vi "sub_qam_demod.vi"(8 "symbol map":cdb[](array[numeric]), 11 "symbol":cdb[](array[numeric])) -> (3 "bitstream":i16[](array[numeric]))   [LabVIEW 2014]
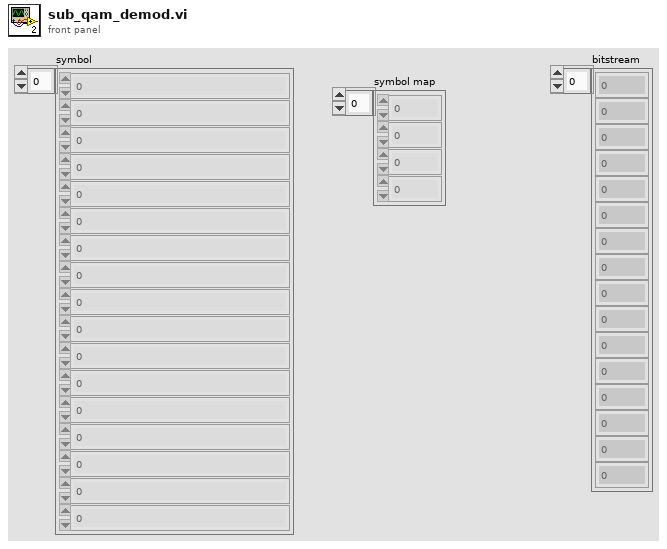
[diagram p1: front panel]
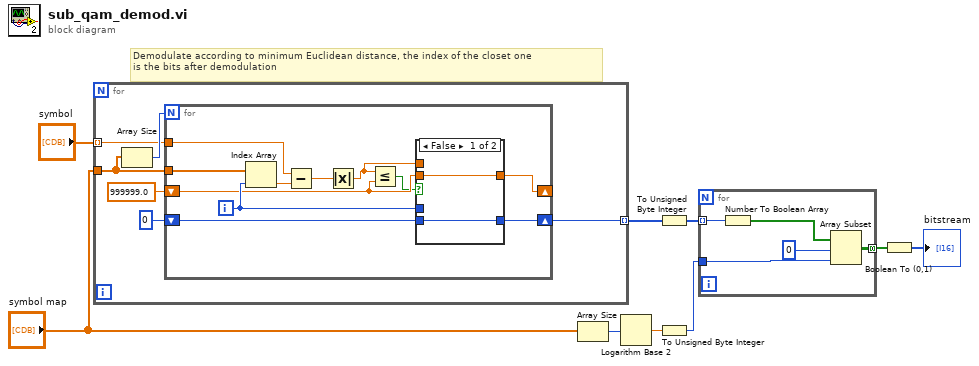
[diagram p0: block diagram]
diagram:
  # "Demodulate according to minimum Euclidean distance, the index of the closet one \nis the bits after demodulation"
  n1 = for {
    tunnel: "symbol map" -> [w14]
    tunnel: "symbol" -> [w13] mode=indexing
    tunnel: [w10] -> w6 mode=indexing
    n2 = Array Size(array=w14) -> (size(s)=w15:i32)
    n3 = for {
      N: w15 -> [_]
      shift-right: [w22] -> _
      shift-left: 999999.0 -> [w17]
      tunnel: w14 -> [w26]
      tunnel: w13 -> [w25]
      shift-right: [w20] -> w10
      shift-left: 0 -> [w19]
      i -> [w21]
      n4 = Index Array(array=w26, index=w21) -> (element=w24:cdb)
      n5 = Subtract(x=w25, y=w24) -> (x-y=w23:cdb)
      n6 = Absolute Value(x=w23) -> (abs(x)=w18:dbl)
      n7 = Less Or Equal?(x=w18, y=w17) -> (x <= y?=w16:bool)
      n8 = case shown="False" w16 {
        tunnel: [w28 w30] -> w22
        tunnel: w18 -> [_ w30]
        tunnel: w21 -> [_ w29]
        tunnel: [w27 w29] -> w20
        tunnel: w17 -> [w28 _]
        tunnel: w19 -> [w27 _]
        frame False {
        }
        frame True {
        }
      }
    }
  }
  n9 = Array Size(array="symbol map") -> (size(s)=w4:i32)
  n10 = Logarithm Base 2(1:w4) -> (0:w3:dbl)
  n11 = To Unsigned Byte Integer(number=w6) -> (unsigned 8bit integer=w8:u8[])
  n12 = To Unsigned Byte Integer(number=w3) -> (unsigned 8bit integer=w2:u8)
  n13 = for {
    tunnel: w8 -> [w35] mode=indexing
    tunnel: w2 -> [w34]
    tunnel: [w32] -> w7 mode=concatenating
    n14 = Number To Boolean Array(number=w35) -> (Boolean array=w31:bool[])
    n15 = Array Subset(array=w31, index=0, length=w34) -> (w32:bool[])
  }
  n16 = Boolean To (0,1)(Boolean=w7) -> (0, 1=→"bitstream":i16[])
